vi "Initialize.vi"(8 "error in":errorcluster, 10 "Root Path":path) -> (0 "error out":errorcluster, 3 "Report Generator out":refnum<class "Report Generator.lvclass">)   [LabVIEW 2018, in "Report Generator.lvlib" / "Report Generator.lvclass"]
uses:
  Report Generator.lvclass
  Report Generator.lvclass/Report Generator.ctl
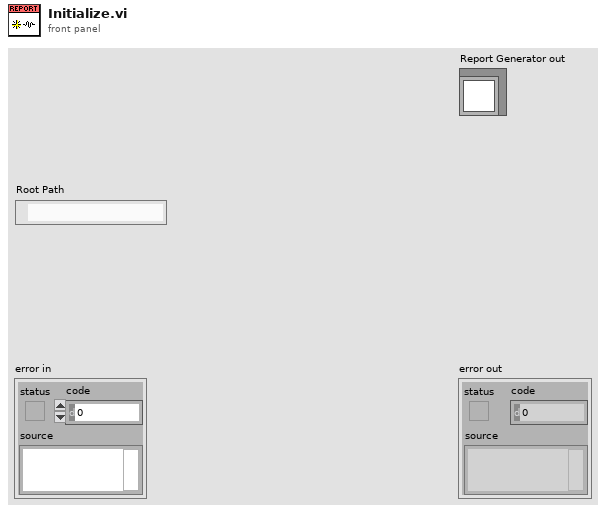
[diagram p1: front panel]
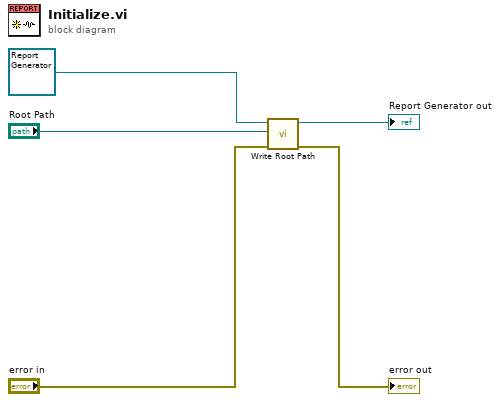
[diagram p0: block diagram]
diagram:
  n1 = call "Write Root Path.vi"("error in (no error)"="error in", "Root Path"="Root Path", "Report Generator in"=refnum<class "Report Generator.lvclass"> refnum) -> ("error out"=→"error out":errorcluster, "Report Generator out"=→"Report Generator out":refnum<class "Report Generator.lvclass">)  [unwired: 7 in]
